vi "MatchDeviceSerialNumber.vi"(8 "error in (no error)":errorcluster, 11 "Serial Number":string) -> (0 "error out":errorcluster, 2 "Match":bool, 3 "BT Serial":T1)   [LabVIEW 2013, in "main.lvlib"]
uses:
  main.lvlib
  Controls/Enum Variables.ctl
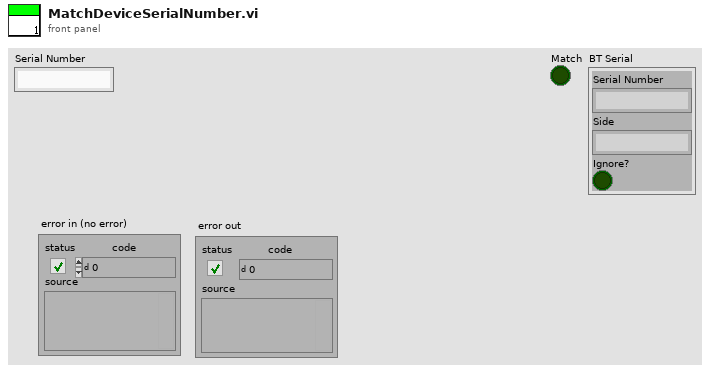
[diagram p1: front panel]
types:
  T1 = cluster{"Serial Number":string, "Side":string, "Ignore?":bool}
  T2 = cluster{"Serial Number":string, "Side":string, "Ignore?":bool}[]
  T3 = typedef "main.lvlib/Enum Variables.ctl" = enum16{"SetAcqFilter", "GetAcqFilter", "Set Filter", "Get Filter", "Set Height", "Get Height", "Set Recorded Height", "Get Recorded Height", "Set Blue Pressure", "Get Blue Pressure", "Set Red Pressure", "Get Red Pressure", "Init", "Reset Pressure", "Set Red Cursors", "Get Red Cursors", "Set Blue Cursors", "Get Blue Cursors", "Set Language", "Get Language", "Set Active Graphs", "Get ActiveGraphs", "Set Method", "Get Method", "Set Encryption", "Get Encryption", "Set ExcelVersion", "Get ExcelVersion", "Set DICOM Avail", "Get DICOM Avail", "Set DICOM Encode", "Get DICOM Encode", "Set JournalExport", "Get JournalExport", "Set Sequence", "Get Sequence", "Set DAQ Connected", "Get DAQ Connected", "Set Current Graph", "Get Current Graph", "Set General Settings", "Get Hyphenation", "Set Arm Calc Method", "Get Arm Calc Method", "Set Dicom Tags", "Get Dicom Tags", "Set BT Serial", "Get BT Serial", "Set BT Accepted Serials", "Get BT Accepted Serials", "Get BT License", "Set BT License"}
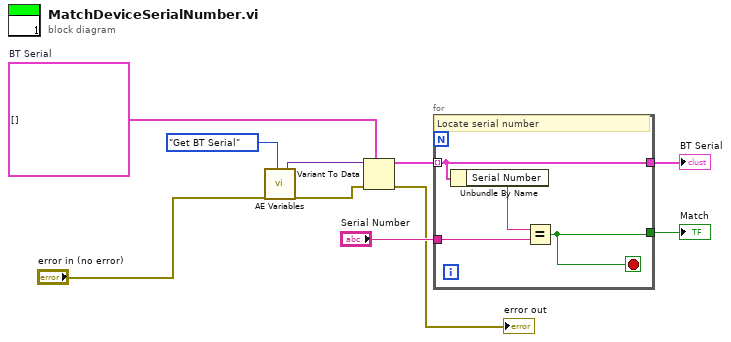
[diagram p0: block diagram]
diagram:
  w10 = T2 []  # BT Serial
  n1 = call "AE Variables.vi"("error in (no error)"="error in (no error)", "Action"=Enum_Variables."Get BT Serial") -> ("Variant"=w9:variant, "error out"=w2:errorcluster)  [unwired: 10 in, 6 out]
  n2 = Variant To Data(error in=w2, type=w10, Variant=w9) -> (data=w7:T2, error out=→"error out":errorcluster)
  n3 = for {
    tunnel: w7 -> [w11] mode=indexing
    tunnel: "Serial Number" -> [w13]
    tunnel: [w12] -> w5
    tunnel: [w11] -> w4
    stop <- w12 stop-if-true
    # "Locate serial number"
    n4 = Unbundle By Name(w11) -> ("Serial Number"=w14:string)
    n5 = Equal?(x=w14, y=w13) -> (x = y?=w12:bool)
  }
  "Match" <- w5
  "BT Serial" <- w4
